vi "testclient.vi"() -> ()   [LabVIEW 2013]
uses:
  <vilib>/Analysis/baseanly.llb/Mean (DBL).vi
  <vilib>/httpClient/LabVIEWHTTPClient.lvlib
  <vilib>/Analysis/NI_AALBase.lvlib
panel:
  out "error out":errorcluster
  in  "Numeric 2":i32=1000
  out "Numeric":dbl
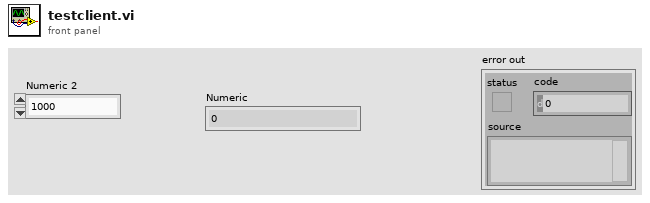
[diagram p1: front panel]
types:
  T1 = typedef "LabVIEWHTTPClient.lvlib/ClientHandle.ctl" = refnum<k1>
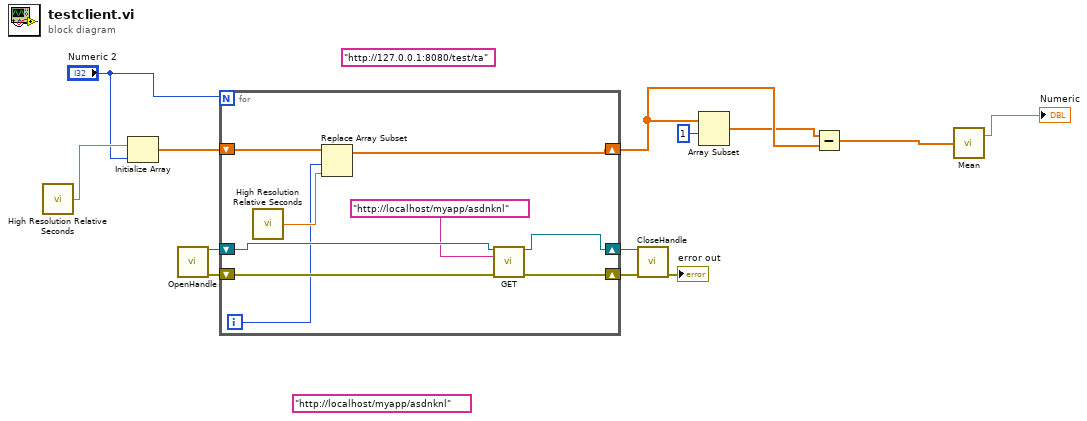
[diagram p0: block diagram]
diagram:
  (unwired) "http://127.0.0.1:8080/test/ta" ("url")
  (unwired) "http://localhost/myapp/asdnknl" ("url")
  n1 = call <vilib>:"High Resolution Relative Seconds.vi"() -> ("relative seconds"=w9:dbl)
  n2 = Initialize Array(w9, "Numeric 2") -> (w7:dbl[])
  n3 = call <vilib>:"OpenHandle.vi"() -> ("client handle out"=w13:T1, "error out"=w11:errorcluster)  [unwired: 14 in]
  n4 = for {
    N: "Numeric 2" -> [_]
    shift-right: [w19] -> w12
    shift-left: w13 -> [w22]
    shift-right: [w20] -> w10
    shift-left: w11 -> [w21]
    shift-right: [w17] -> w6
    shift-left: w7 -> [w18]
    i -> [w15]
    n5 = call <vilib>:"High Resolution Relative Seconds.vi"() -> ("relative seconds"=w16:dbl)
    n6 = Replace Array Subset(array=w18, new element=w16, index=w15) -> (w17:dbl[])
    n7 = call <vilib>:"GET.vi"("client handle"=w22, "url"="http://localhost/myapp/asdnknl", "error in (no error)"=w21) -> ("client handle out"=w19:T1, "error out"=w20:errorcluster)  [unwired: 9 in, 2 out]
  }
  n8 = call <vilib>:"CloseHandle.vi"("client handle"=w12, "error in (no error)"=w10) -> ("error out"=→"error out":errorcluster)  [unwired: 13 in]
  n9 = Array Subset(array=w6, index=1) -> (w4:dbl[])  [unwired: 1 in]
  n10 = Subtract(x=w4, y=w6) -> (x-y=w3:dbl[])
  n11 = call-poly <vilib>:"Mean.vi"("X"=w3) -> ("mean"=→"Numeric":dbl)  [unwired: 1 out]
